vi "ClassAppData.Set.vi"(7 "Section":string, 8 "error in (no error)":errorcluster, 9 "Value":variant, 10 "Name":string, 11 "Class - App Data in":refnum<class "Class.AppData.lvclass">) -> (0 "error out":errorcluster, 2 "Replaced":bool, 3 "Class - App Data out":refnum<class "Class.AppData.lvclass">)   [LabVIEW 2024, in "EQMF.lvlib" / "Config Utils.lvlib" / "Class.AppData.lvclass"]
doc: "<B>AppData Class:</B>\nThe AppData class keeps track of a library of data items that are used by an application. These data items have a name (text string) and value that can be any data type. \n\nThis VI is part of the AppData class. This VI will add or update the AppData item specified by the Section and Name input. \n\nINPUTS:\n<B>Section and Name</B> - The section and name inputs are used to build the name of the item to be set. If only the Name input is populated, then that will be used for the name of the item to set. If both are populated the then the Section and Name will be concatenated with a period separator and that will be used for the name of the item to set.\nEXAMPLE: If Section = \"AA\" and Name = \"BB\" then the name used for the data item will be \"AA.BB\".\n<B>Value</B> - This is a variant containing the value of the item to be set.\n\nOUTPUTS:\n<B>Replaced</B> - This is TRUE if the item existed in the library and its value was updated. This is FALSE if the item did not exist and it was added to the library."
uses:
  Class.AppData.lvclass
  Class.AppData.lvclass/Class.AppData.ctl
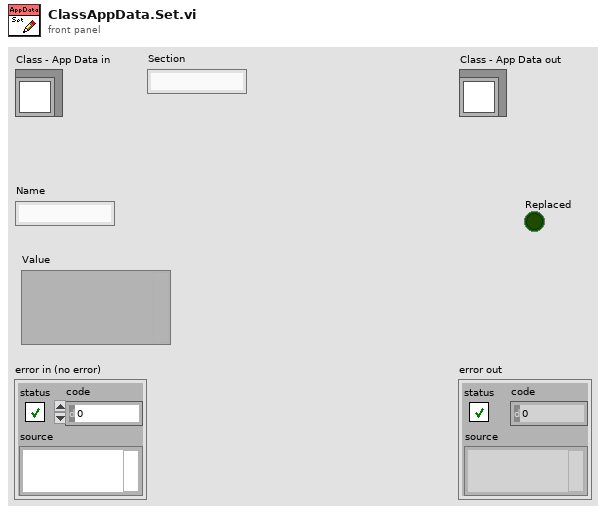
[diagram p1: front panel]
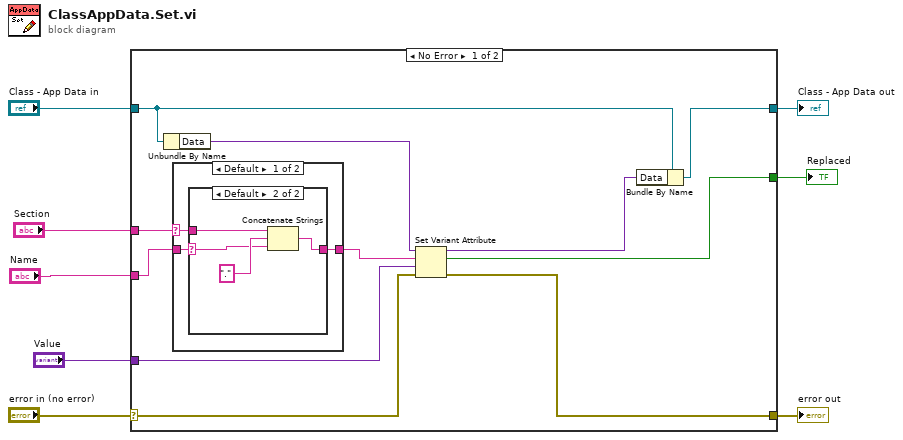
[diagram p0: block diagram]
diagram:
  n1 = case shown="No Error" "error in (no error)" {
    selector: "error in (no error)" -> [w18 w30]
    tunnel: [w17 w30] -> w7
    tunnel: [w15 w29] -> w5
    tunnel: "Class - App Data in" -> [w16 w29]
    tunnel: [w13 _] -> w4
    tunnel: "Value" -> [w12 _]
    tunnel: "Name" -> [w10 _]
    tunnel: "Section" -> [w11 _]
    frame No Error {
      n2 = Unbundle By Name(w16) -> ("Data"=w19:variant)
      n3 = case shown="Default" w11 {
        selector: w11 -> [w22 _]
        tunnel: w10 -> [w20 w28]
        tunnel: [w21 w28] -> w9
        frame Default {
          n4 = case shown="Default" w20 {
            selector: w20 -> [_ w24]
            tunnel: w22 -> [w23 w27]
            tunnel: [w23 w25] -> w21
            frame "" {
            }
            frame Default {
              n5 = Concatenate Strings(w27, ".", w24) -> (w25:string)
            }
          }
        }
        frame "" {
        }
      }
      n6 = Set Variant Attribute(Variant=w19, name=w9, value=w12, error in=w18) -> (Variant out=w14:variant, replaced=w13:bool, error out=w17:errorcluster)
      n7 = Bundle By Name(cluster=w16, "Data"=w14) -> (w15:refnum<class "Class.AppData.lvclass">)
    }
    frame Error {
    }
  }
  "error out" <- w7
  "Class - App Data out" <- w5
  "Replaced" <- w4
